vi "CloseDevices.vi"(8 "error in (no error)":errorcluster, 11 "Ids":i32[](array[numeric])) -> (0 "error out":errorcluster)   [LabVIEW 2020]
uses:
  libximc.lvlib
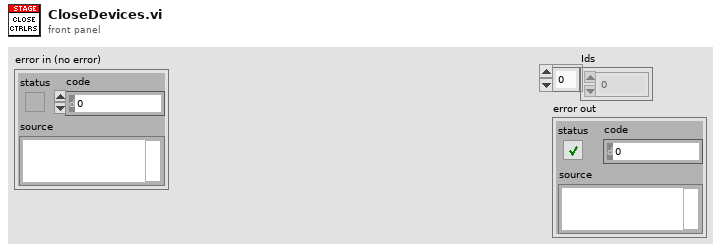
[diagram p1: front panel]
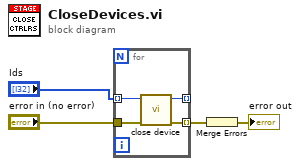
[diagram p0: block diagram]
diagram:
  n1 = for {
    tunnel: [w8] -> _ mode=indexing
    tunnel: "Ids" -> [w7] mode=indexing
    tunnel: "error in (no error)" -> [w6]
    tunnel: [w5] -> w2 mode=indexing
    n2 = call "close device.vi"("error in (no error)"=w6, "id"=w7) -> ("error out"=w5:errorcluster, "id out"=w8:i32)  [unwired: 7 in, 1 out]
  }
  n3 = Merge Errors(w2) -> (→"error out":errorcluster)
